vi "ChangePassword-Window.vi"(7 "PwdMgr":refnum<class "PwdMgr.lvclass">, 8 "error in (no error)":errorcluster, 11 "User Info":T1={"UserName"="", "Password"="", "Role"=enum."Admin"}) -> (0 "error out":errorcluster)   [LabVIEW 2020, in "Login-UI.lvlib"]
uses:
  Login-UI.lvlib
  _Typedef/User-Info.ctl
  _Typedef/User-Role.ctl
  PwdMgr/PwdMgr.lvclass
panel:
  in  "Exit":bool
  in  "Save":bool
  in  "密  码":string
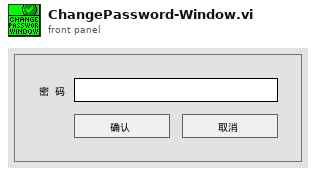
[diagram p1: front panel]
types:
  T1 = typedef "Login-UI.lvlib/User-Info.ctl" = cluster{"UserName":string, "Password":string, "Role":T2}
  T2 = typedef "Login-UI.lvlib/User-Role.ctl" = enum16{"INVALID", "Operator", "Engineer", "Admin", "Anonymous"}
  T3 = enum32{"Invalid", "Standard", "Closed", "Hidden", "Minimized", "Maximized"}
  T4 = enum32{"invalid app kind", "Development System", "Run Time System", "Student Edition", "Embedded LabVIEW", "Evaluation", "Custom"}
  T5 = cluster{"Core":cluster{"Current VI Reference":refnum<vi>, "Close Panel on Exit?":bool}, "Your Boolean data":bool, "Your string data":string, "User Info":T1}
  T6 = typedef "eventvkey.ctl" = enum16{"ASCII", "Enter", "Return", "Shift", "Ctrl", "Alt", "Cmd", "Opt", "Caps", "NumLock", "Clear", "Break", "Up", "Down", "Left", "Right", "Insert", "Delete", "Home", "End", "PageUp", "PageDown", "Escape", "Help", "Pause", "ScrollLock", "F1", "F2", "F3", "F4", "F5", "F6", "F7", "F8", "F9", "F10", "F11", "F12", "F13", "F14", "F15", "F16", "F17", "F18", "F19", "F20", "F21", "F22", "F23", "F24", "Play", "VolumeUp", "VolumeDown", "Mute", "Two Byte Char"}
  T7 = cluster{"Current VI Reference":refnum<vi>, "Close Panel on Exit?":bool}
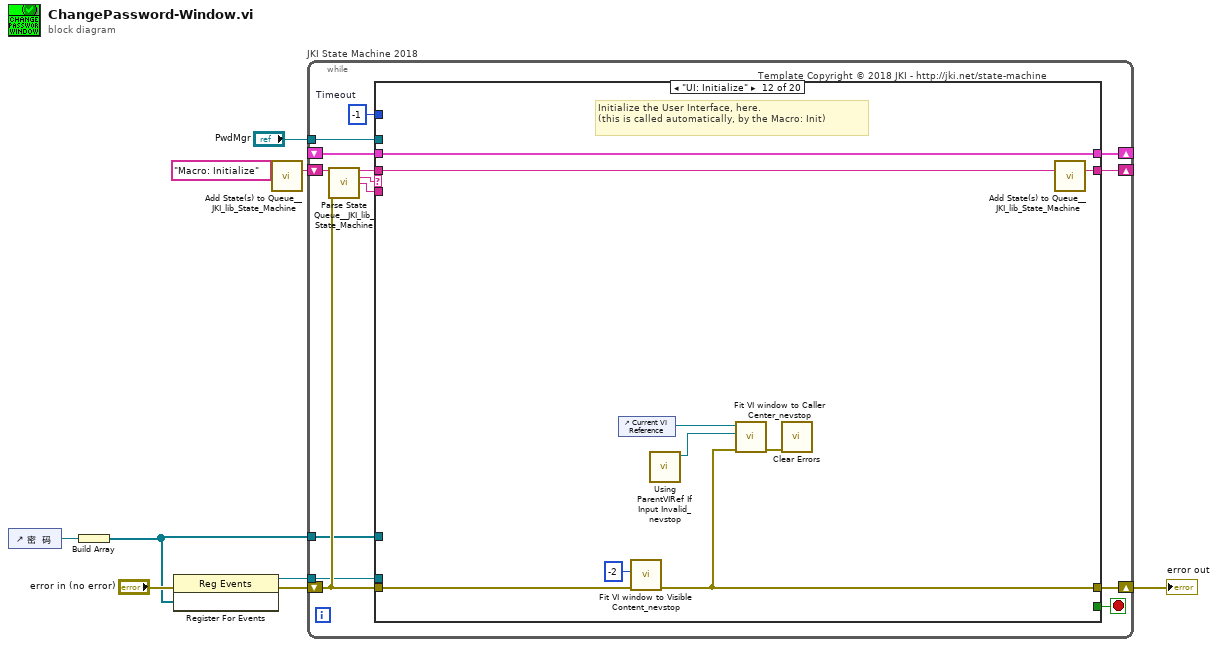
[diagram p0: block diagram]
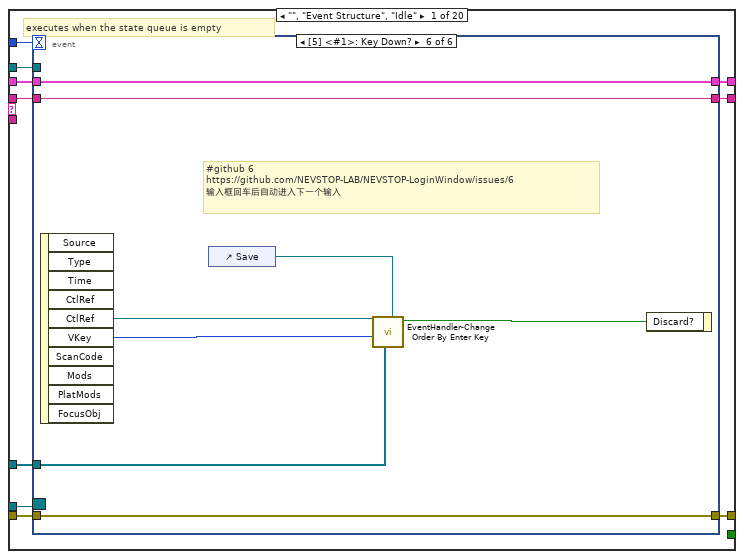
[diagram p2: hidden frame]
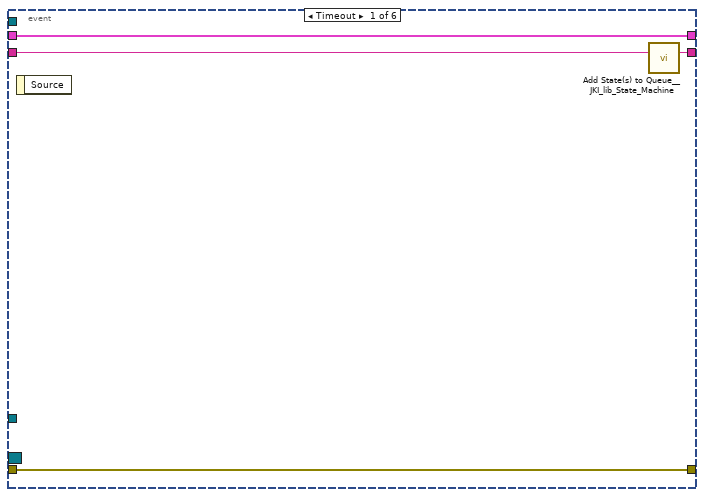
[diagram p3: hidden frame]
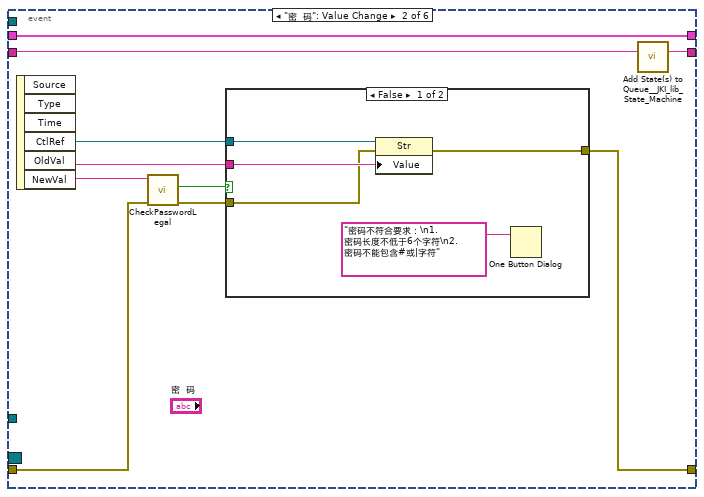
[diagram p4: hidden frame]
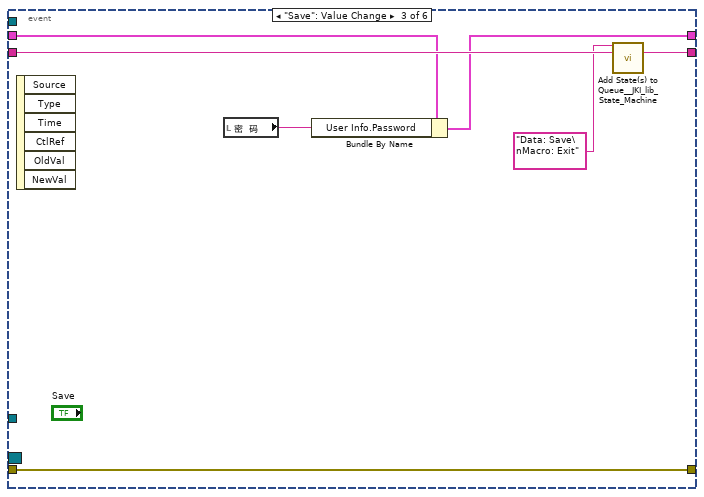
[diagram p6: hidden frame]
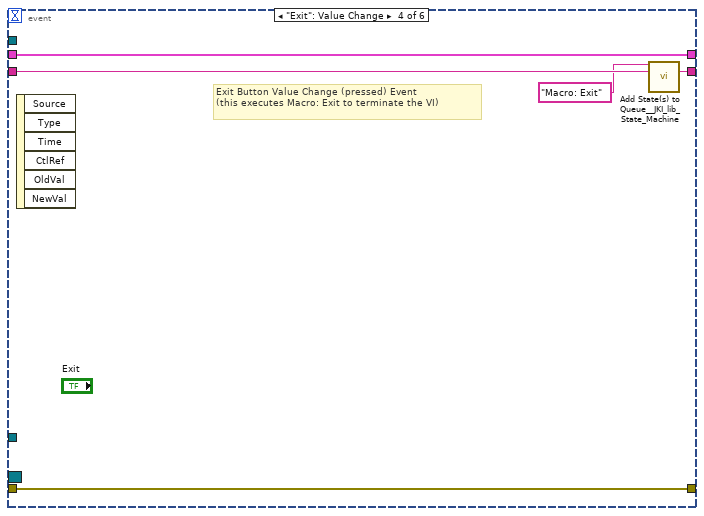
[diagram p7: hidden frame]
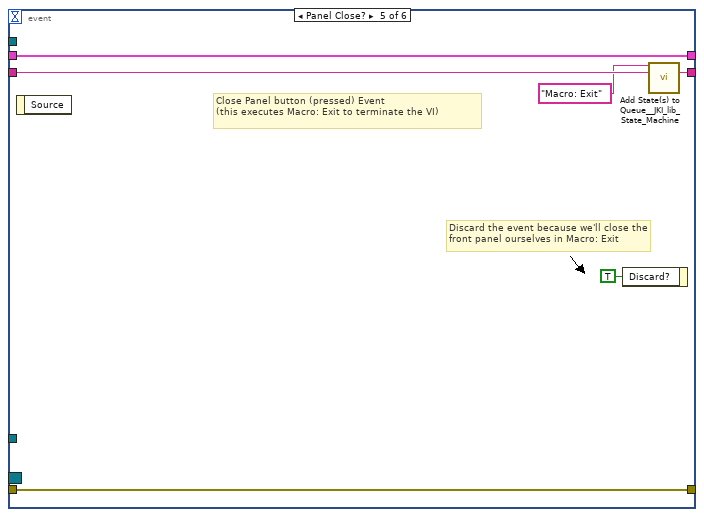
[diagram p8: hidden frame]
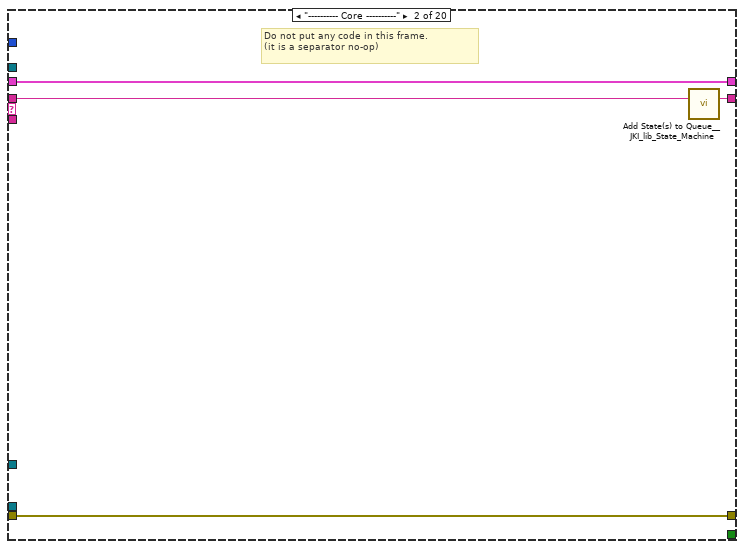
[diagram p9: hidden frame]
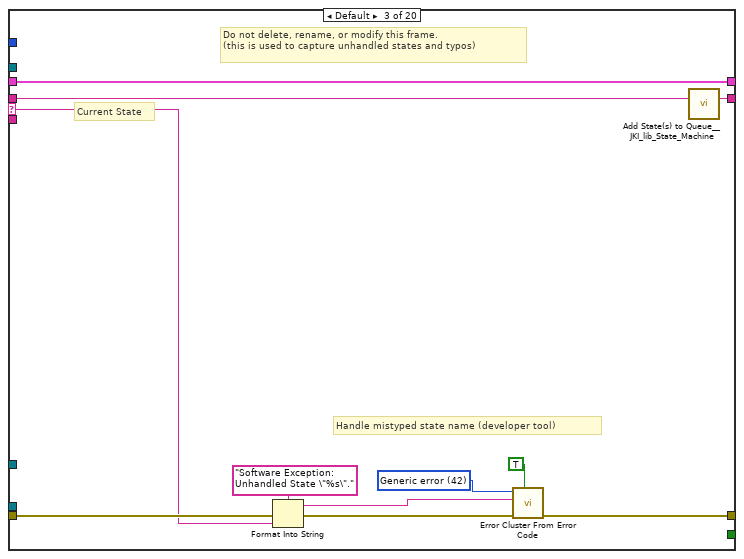
[diagram p10: hidden frame]
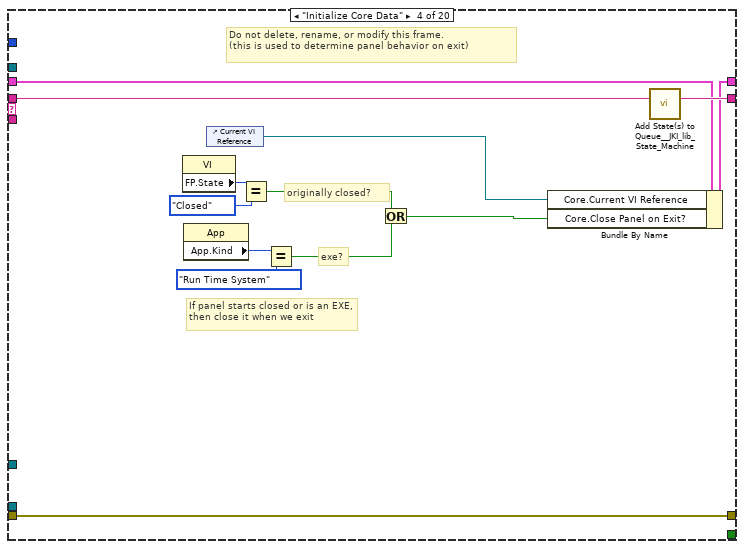
[diagram p11: hidden frame]
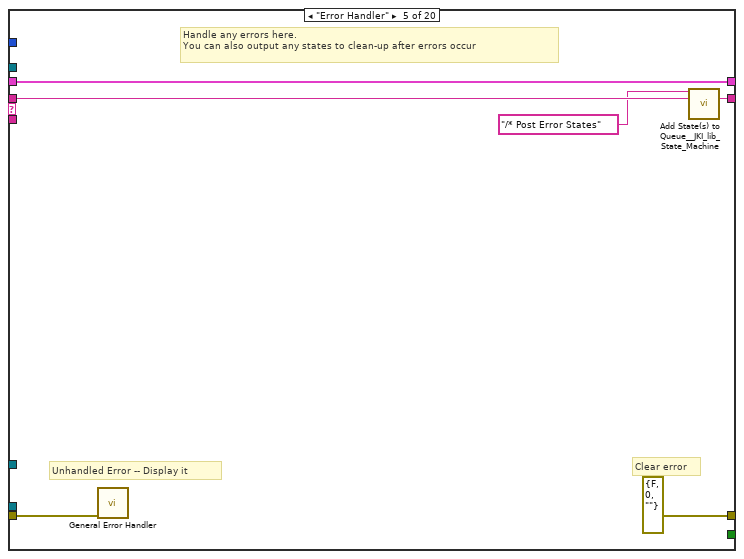
[diagram p12: hidden frame]
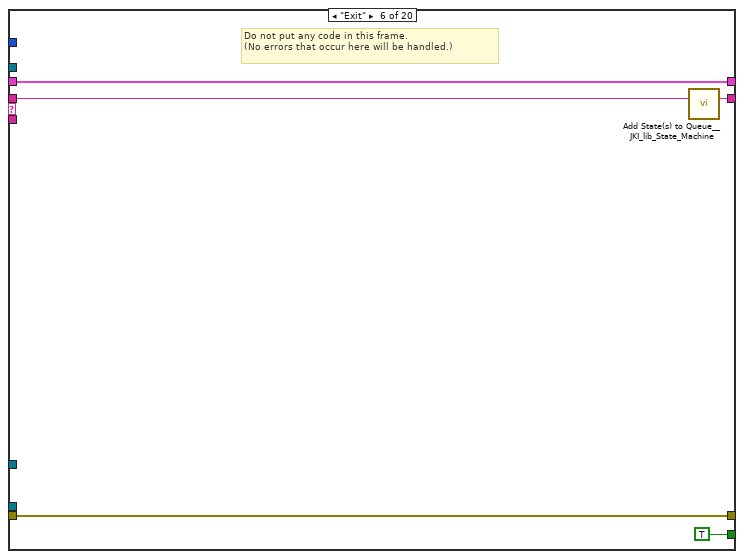
[diagram p13: hidden frame]
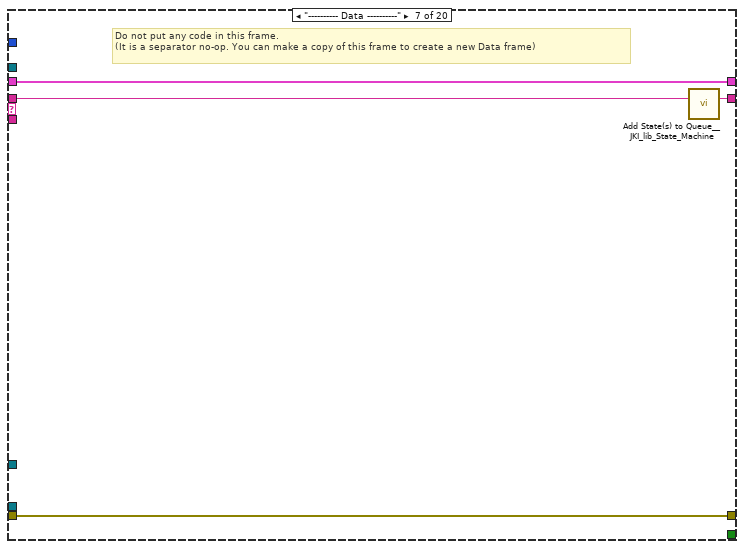
[diagram p14: hidden frame]
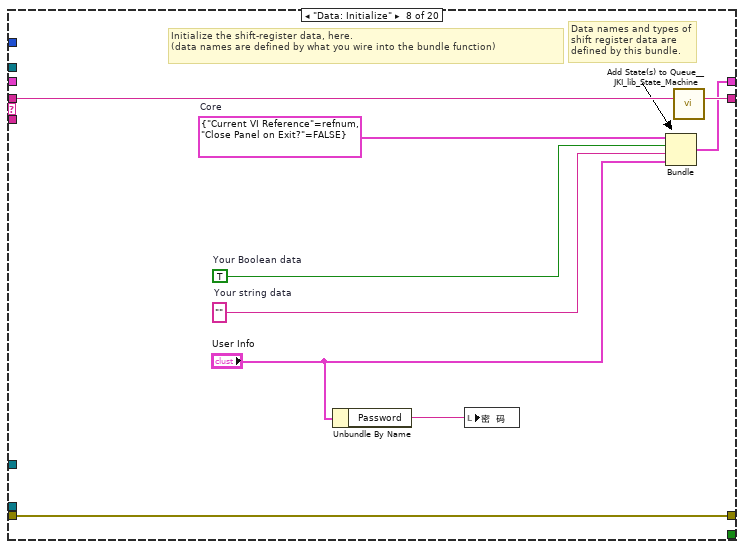
[diagram p15: hidden frame]
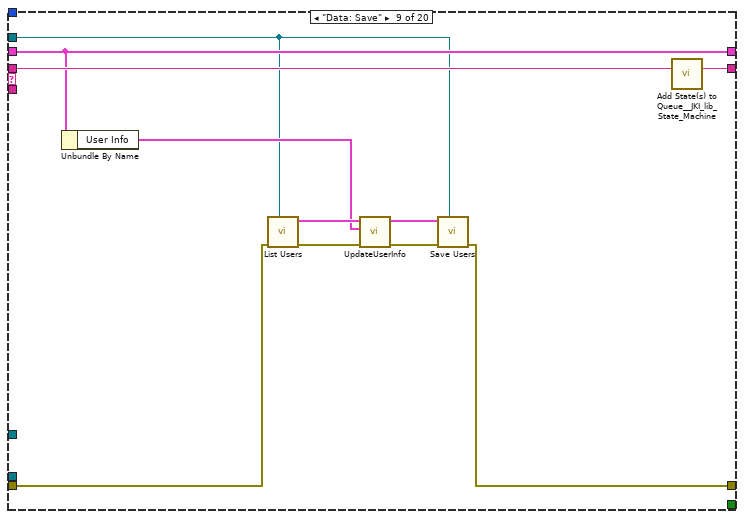
[diagram p16: hidden frame]
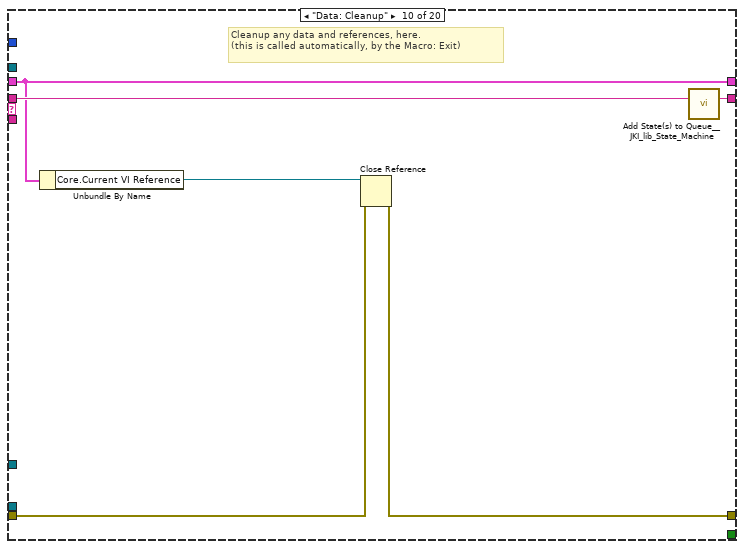
[diagram p17: hidden frame]
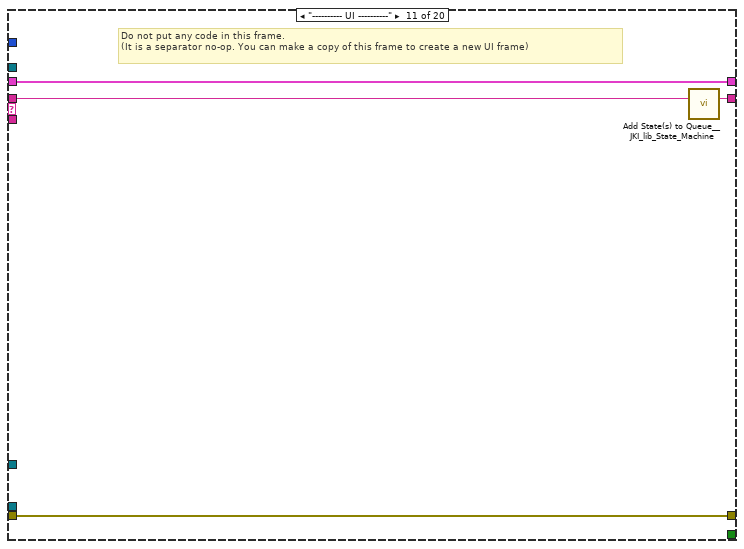
[diagram p18: hidden frame]
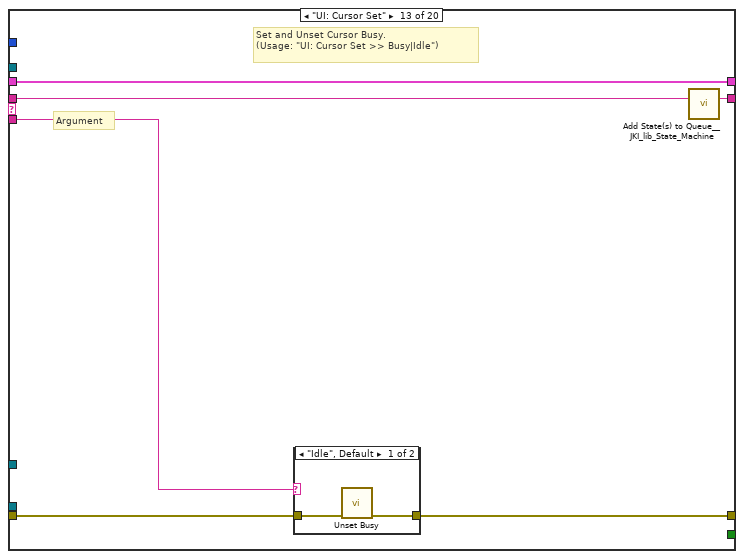
[diagram p19: hidden frame]
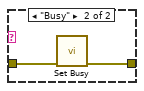
[diagram p20: hidden frame]
diagram:
  n1 = control-ref of="密  码"() -> (w3:refnum<vi>)
  n2 = Build Array(w3) -> (w2:refnum<vi>[])
  n3 = register-events(error in="error in (no error)", w2) -> (reference out=w4:refnum<event-registration>, error out=w5:errorcluster)  [unwired: 1 in]
  n4 = call <vilib>:"Add State(s) to Queue__JKI_lib_State_Machine.vi"("State(s) in (\"\")"="Macro: Initialize") -> ("States Out"=w9:string)  [unwired: 14 in]
  n5 = while "JKI State Machine 2018" {
    shift-right: [w16] -> _
    shift-left: _ -> [w15]
    shift-right: [w19] -> w6
    shift-left: w5 -> [w13]
    shift-right: [w18] -> _
    shift-left: w9 -> [w20]
    tunnel: w4 -> [w12]
    tunnel: w2 -> [w11]
    tunnel: "PwdMgr" -> [w10]
    stop <- w17 stop-if-true
    w14 = -1  # Timeout
    # "Template Copyright © 2018 JKI - http://jki.net/state-machine"
    n6 = call <vilib>:"Parse State Queue__JKI_lib_State_Machine.vi"("State Queue"=w20, "Error In (no error)"=w13) -> ("Remaining States"=w22:string, "Current State"=w23:string, "Arguments"=w21:string)  [unwired: 11 in]
    n7 = case shown="\"UI: Initialize\"" w23 {
      selector: w23 -> [_ _ w84 _ _ _ _ _ _ _ _ _ _ _ _ _ _ _ _ _]
      tunnel: w22 -> [w33 w83 w88 w107 w113 w118 w122 w131 w141 w148 w152 w161 w167 w178 w247 w252 w262 w266 w270 w274]
      tunnel: w21 -> [_ _ _ _ _ _ _ _ _ _ _ _ w162 w172 _ _ _ _ _ _]
      tunnel: w15 -> [w31 w80 w86 w100 w110 w116 w119 _ w133 w143 w149 w159 w165 w174 w244 w249 w259 w263 w267 w271]
      tunnel: [w30 w81 w90 w104 errorcluster {"status"=FALSE, "code"=0, "source"=""} ("error out") w115 w120 w128 w134 w144 w150 w153 w163 w175 w245 w250 w260 w264 w268 w272] -> w19
      tunnel: w13 -> [w29 w81 w89 w104 w109 w115 w120 w128 w135 w145 w150 w157 w164 w176 w245 w250 w260 w264 w268 w272]
      tunnel: [w32 w82 w87 w106 w112 w117 w121 w130 w142 w147 w151 w160 w166 w177 w246 w251 w261 w265 w269 w273] -> w18
      tunnel: [_ _ _ _ _ TRUE _ _ _ _ _ _ _ _ _ _ _ _ _ _] -> w17
      tunnel: [w28 w80 w86 w105 w110 w116 w119 w129 w133 w143 w149 w159 w165 w174 w244 w249 w259 w263 w267 w271] -> w16
      tunnel: w14 -> [w27 _ _ _ _ _ _ _ _ _ _ _ _ _ _ _ _ _ _ _]
      tunnel: w12 -> [w26 _ _ _ _ _ _ _ _ _ _ _ _ _ _ _ _ _ _ _]
      tunnel: w11 -> [w25 _ _ _ _ _ _ _ _ _ _ _ _ _ _ _ _ _ _ _]
      tunnel: w10 -> [w24 _ _ _ _ _ _ _ w132 _ _ _ _ _ _ _ _ _ _ _]
      frame "", "Event Structure", "Idle" {
        # "executes when the state queue is empty"
        n8 = event shown="[5] <#1>: Key Down?" {
          selector: w26 -> [_ _ _ _ _ _]
          dyn-events: _ -> [_ _ _ _ _ _]
          timeout: w27 -> [_ _ _ _ _ _]
          tunnel: w33 -> [w37 w41 w59 w65 w71 w73]
          tunnel: [w36 w42 w60 w64 w70 w73] -> w32
          tunnel: w31 -> [w34 w43 w57 w62 w68 w74]
          tunnel: [w35 w38 w55 w63 w69 w72] -> w30
          tunnel: w29 -> [w35 w40 w55 w63 w69 w72]
          tunnel: [w34 w43 w56 w62 w68 w74] -> w28
          tunnel: w25 -> [_ _ _ _ _ w76]
          tunnel: w24 -> [_ _ _ _ _ _]
          event Timeout {
            n9 = event-data() -> ()  [unwired: 1 in, 1 out]
            n10 = call <vilib>:"Add State(s) to Queue__JKI_lib_State_Machine.vi"("State(s) in (\"\")"=w37) -> ("States Out"=w36:string)  [unwired: 14 in]
          }
          event "密  码": Value Change {
            n11 = event-data() -> ("CtlRef"=w45:refnum<vi>, "OldVal"=w44:string, "NewVal"=w47:string)  [unwired: 1 in, 3 out]
            n12 = call "CheckPasswordLegal.vi"("error in (no error)"=w40, "Password"=w47) -> ("error out"=w39:errorcluster, "legal?"=w46:bool)  [unwired: 8 in]
            n13 = case shown="False" w46 {
              tunnel: w45 -> [w52 _]
              tunnel: w44 -> [w51 _]
              tunnel: w39 -> [w49 w53]
              tunnel: [w48 w53] -> w38
              frame False {
                n14 = property class="Str"(reference=w52, error in=w49, "Value"=w51) -> (error out=w48:errorcluster)  [unwired: 1 out]
                n15 = One Button Dialog(message="密码不符合要求：\n1.密码长度不低于6个字符\n2. 密码不能包含#或|字符") -> ()  [unwired: 1 in, 1 out]
              }
              frame True {
              }
            }
            n16 = call <vilib>:"Add State(s) to Queue__JKI_lib_State_Machine.vi"("State(s) in (\"\")"=w41) -> ("States Out"=w42:string)  [unwired: 14 in]
          }
          event "Save": Value Change {
            n17 = event-data() -> ()  [unwired: 1 in, 6 out]
            n18 = local read "密  码"() -> (w54:string)
            n19 = Bundle By Name(cluster=w57, "User Info.Password"=w54) -> (w56:T5)
            n20 = call <vilib>:"Add State(s) to Queue__JKI_lib_State_Machine.vi"("State(s) in Front (\"\")"="Data: Save\nMacro: Exit", "State(s) in (\"\")"=w59) -> ("States Out"=w60:string)  [unwired: 13 in]
          }
          event "Exit": Value Change {
            # "Exit Button Value Change (pressed) Event\n(this executes Macro: Exit to terminate the VI)"
            n21 = event-data() -> ()  [unwired: 1 in, 6 out]
            n22 = call <vilib>:"Add State(s) to Queue__JKI_lib_State_Machine.vi"("State(s) in Front (\"\")"="Macro: Exit", "State(s) in (\"\")"=w65) -> ("States Out"=w64:string)  [unwired: 13 in]
          }
          event Panel Close? {
            # "Discard the event because we'll close the front panel ourselves in Macro: Exit"
            # "Close Panel button (pressed) Event\n(this executes Macro: Exit to terminate the VI)"
            n23 = event-data() -> ()  [unwired: 1 in, 1 out]
            n24 = event-data("Discard?"=TRUE) -> ()  [unwired: 1 in, 1 out]
            n25 = call <vilib>:"Add State(s) to Queue__JKI_lib_State_Machine.vi"("State(s) in Front (\"\")"="Macro: Exit", "State(s) in (\"\")"=w71) -> ("States Out"=w70:string)  [unwired: 13 in]
          }
          event Key Down? {
            # "#github 6\nhttps://github.com/NEVSTOP-LAB/NEVSTOP-LoginWindow/issues/6\n输入框回车后自动进入下一个输入"
            n26 = event-data() -> ("CtlRef"=w79:refnum<vi>, "VKey"=w78:T6)  [unwired: 1 in, 8 out]
            n27 = control-ref of="Save"() -> (w77:refnum<vi>)
            n28 = call "EventHandler-Change Order By Enter Key.vi"("Next Ctrl"=w77, "Controls for changing order"=w76, "VKey"=w78, "Event Control"=w79) -> ("Discard?"=w75:bool)  [unwired: 7 in]
            n29 = event-data("Discard?"=w75) -> ()  [unwired: 1 in, 1 out]
          }
        }
      }
      frame "---------- Core ----------" {
        # "Do not put any code in this frame.\n(it is a separator no-op)"
        n30 = call <vilib>:"Add State(s) to Queue__JKI_lib_State_Machine.vi"("State(s) in (\"\")"=w83) -> ("States Out"=w82:string)  [unwired: 14 in]
      }
      frame Default {
        w93 = 42 items=["No error", "Argument error", "Memory is full", "Out of zone", "End of file", "File already open", "Generic file I/O error", "File not found", "File permission error", "Disk is full", "Duplicate path", "Too many files open", "System feature not enabled", "Resource file not found", "Cannot add resource", "Resource not found", "Image not found", "Image memory error", "Pen does not exist", "Config type invalid", "Config token not found", "Config parse error", "Config memory error", "Bad external code format", "Bad external code offset", "External code not present", "Null window", "Destroy window error", "Null menu", "Print aborted", "Bad print record", "Print driver error", "Windows error during printing", "Memory error during printing", "Print dialog error", "Generic print error", "Invalid device refnum", "Device not found", "Device parameter error", "Device unit error", "Cannot open device", "Device call aborted", "Generic error", "Cancelled by user", "Object ID too low", "Object ID too high", "Object not in heap", "Unknown heap", "Unknown object (invalid DefProc)", "Unknown object (DefProc not in table)", "Message out of range", "Invalid (null) method", "Unknown message", "Manager call not supported", "Bad address", "Network operation in progress", "Network operation timed out", "Connection is busy", "Network attribute not supported", "Network error", "Address in use", "System out of memory", "Connection aborted", "Connection refused", "Not connected", "Already connected", "Connection closed", "Initialization error (interapplication manager)", "Bad occurrence", "Wait on unbound occurrence handler", "Occurrence queue overflow", "Datalog type conflict", "Unused", "Unrecognized type (interapplication manager)", "Memory corrupt", "Failed to make temporary DLL", "Old CIN version", "Drag socket not found", "Failed to load drop-object", "Failed to register OLE object", "Failed to release OLE object", "Format specifier type mismatch", "Unknown format specifier", "Too few format specifiers", "Too many format specifiers", "Scan failed", "Newer CIN version", "Error converting to variant", "Runtime menu error", "Password tampered", "Variant attribute not found", "Incompatible variant data type", "Event data is not available", "Event Store is not present", "Occurrence is not found", "Event Queue is not created", "Event info is not available", "Refnum passed is NULL", "Error retrieving Class GUID", "Error retrieving CoClass GUID", "Error retrieving TypeLib GUID.", "Bad built application magic bytes.", "Specific driver is different from the specific driver associated with the Logical Name.", "There is no session opened to the class driver.", "Max Error", "MAX - Error with config objects", "MAX - Error loading configuration", "MAX - Group not supported"]
        # "Current State"
        # "Do not delete, rename, or modify this frame.\n(this is used to capture unhandled states and typos)"
        # "Handle mistyped state name (developer tool)"
        n31 = Format Into String(format string="Software Exception: Unhandled State \"%s\"." ("message"), error in=w89, w84) -> (resulting string=w92:string, error out=w91:errorcluster)  [unwired: 1 in]
        n32 = call <vilib>:"Error Cluster From Error Code.vi"("show call chain? (False)"=TRUE, "error in (no error)"=w91, "error message (\"\")"=w92, "error code (0)"=w93) -> ("error out"=w90:errorcluster)  [unwired: 5 in]
        n33 = call <vilib>:"Add State(s) to Queue__JKI_lib_State_Machine.vi"("State(s) in (\"\")"=w88) -> ("States Out"=w87:string)  [unwired: 14 in]
      }
      frame "Initialize Core Data" {
        # "Do not delete, rename, or modify this frame.\n(this is used to determine panel behavior on exit)"
        # "originally closed?"
        # "exe?"
        # "If panel starts closed or is an EXE, then close it when we exit"
        n34 = property class="VI"() -> ("FP.State"=w97:T3)  [unwired: 2 in, 2 out]
        n35 = property class="App"() -> ("App.Kind"=w103:T4)  [unwired: 2 in, 2 out]
        n36 = control-ref of="Current VI Reference"() -> (w98:refnum<vi>)
        n37 = Equal?(x=w97, y=T3."Closed" ("Front Panel Window:State")) -> (x = y?=w95:bool)
        n38 = Equal?(x=w103, y=T4."Run Time System" ("Application:Kind")) -> (x = y?=w101:bool)
        n39 = Or(x=w95, y=w101) -> (x .or. y?=w99:bool)
        n40 = Bundle By Name(cluster=w100, "Core.Current VI Reference"=w98, "Core.Close Panel on Exit?"=w99) -> (w105:T5)
        n41 = call <vilib>:"Add State(s) to Queue__JKI_lib_State_Machine.vi"("State(s) in (\"\")"=w107) -> ("States Out"=w106:string)  [unwired: 14 in]
      }
      frame "Error Handler" {
        # "Unhandled Error -- Display it"
        # "Handle any errors here.\nYou can also output any states to clean-up after errors occur"
        # "Clear error"
        n42 = call <vilib>:"General Error Handler.vi"("error in (no error)"=w109) -> ()  [unwired: 10 in, 5 out]
        n43 = call <vilib>:"Add State(s) to Queue__JKI_lib_State_Machine.vi"("State(s) in Front (\"\")"="/* Post Error States", "State(s) in (\"\")"=w113) -> ("States Out"=w112:string)  [unwired: 13 in]
      }
      frame "Exit" {
        # "Do not put any code in this frame.\n(No errors that occur here will be handled.)"
        n44 = call <vilib>:"Add State(s) to Queue__JKI_lib_State_Machine.vi"("State(s) in (\"\")"=w118) -> ("States Out"=w117:string)  [unwired: 14 in]
      }
      frame "---------- Data ----------" {
        # "Do not put any code in this frame.\n(It is a separator no-op. You can make a copy of this frame to create a new Data frame)"
        n45 = call <vilib>:"Add State(s) to Queue__JKI_lib_State_Machine.vi"("State(s) in (\"\")"=w122) -> ("States Out"=w121:string)  [unwired: 14 in]
      }
      frame "Data: Initialize" {
        w125 = T7 {"Current VI Reference"=refnum, "Close Panel on Exit?"=FALSE}  # Core
        w127 = TRUE  # Your Boolean data
        w126 = ""  # Your string data
        # "Data names and types of shift register data are defined by this bundle."
        # "Initialize the shift-register data, here.\n(data names are defined by what you wire into the bundle function)"
        n46 = Unbundle By Name("User Info") -> ("Password"=w123:string)
        n47 = local write "密  码"(w123) -> ()
        n48 = Bundle("Core"=w125, "Your Boolean data"=w127, "Your string data"=w126, "User Info"="User Info") -> (w129:T5)  [unwired: 1 in]
        n49 = call <vilib>:"Add State(s) to Queue__JKI_lib_State_Machine.vi"("State(s) in (\"\")"=w131) -> ("States Out"=w130:string)  [unwired: 14 in]
      }
      frame "Data: Save" {
        n50 = Unbundle By Name(w133) -> ("User Info"=w139:T1)
        n51 = call-dynamic "List Users.vi"("PwdMgr in"=w132, "error in (no error)"=w135) -> ("error out"=w138:errorcluster, "Array"=w140:T1[])  [unwired: 8 in]
        n52 = call "UpdateUserInfo.vi"("error in"=w138, "User"=w139, "User List"=w140) -> ("error out"=w136:errorcluster, "User List"=w137:T1[])  [unwired: 7 in]
        n53 = call-dynamic "Save Users.vi"("PwdMgr in"=w132, "error in (no error)"=w136, "Array"=w137) -> ("error out"=w134:errorcluster)  [unwired: 8 in]
        n54 = call <vilib>:"Add State(s) to Queue__JKI_lib_State_Machine.vi"("State(s) in (\"\")"=w141) -> ("States Out"=w142:string)  [unwired: 14 in]
      }
      frame "Data: Cleanup" {
        # "Cleanup any data and references, here.\n(this is called automatically, by the Macro: Exit)"
        n55 = Unbundle By Name(w143) -> ("Core.Current VI Reference"=w146:refnum<vi>)
        n56 = Close Reference(reference=w146, error in (no error)=w145) -> (error out=w144:errorcluster)
        n57 = call <vilib>:"Add State(s) to Queue__JKI_lib_State_Machine.vi"("State(s) in (\"\")"=w148) -> ("States Out"=w147:string)  [unwired: 14 in]
      }
      frame "---------- UI ----------" {
        # "Do not put any code in this frame.\n(It is a separator no-op. You can make a copy of this frame to create a new UI frame)"
        n58 = call <vilib>:"Add State(s) to Queue__JKI_lib_State_Machine.vi"("State(s) in (\"\")"=w152) -> ("States Out"=w151:string)  [unwired: 14 in]
      }
      frame "UI: Initialize" {
        # "Initialize the User Interface, here.\n(this is called automatically, by the Macro: Init)"
        n59 = control-ref of="Current VI Reference"() -> (w155:refnum<vi>)
        n60 = call <userlib>:"Fit VI window to Visible Content_nevstop.vi"("error in (no error)"=w157, "border spacing (2 px)"=-2) -> ("error out"=w153:errorcluster)  [unwired: 4 in, 1 out]
        n61 = call <userlib>:"Using ParentVIRef If Input Invalid_nevstop.vi"() -> ("VI Ref"=w154:refnum<vi>)  [unwired: 6 in, 1 out]
        n62 = call <userlib>:"Fit VI window to Caller Center_nevstop.vi"("Error In"=w153, "Background VI Ref (Callee's Caller)"=w154, "VI Ref (calling VI)"=w155) -> ("Error Out"=w156:errorcluster)  [unwired: 3 in, 1 out]
        n63 = call <vilib>:"Clear Errors.vi"("error in (no error)"=w156) -> ()  [unwired: 5 in, 2 out]
        n64 = call <vilib>:"Add State(s) to Queue__JKI_lib_State_Machine.vi"("State(s) in (\"\")"=w161) -> ("States Out"=w160:string)  [unwired: 14 in]
      }
      frame "UI: Cursor Set" {
        # "Argument"
        # "Set and Unset Cursor Busy.\n(Usage: \"UI: Cursor Set >> Busy|Idle\")"
        n65 = case shown="\"Idle\", Default" w162 {
          tunnel: w164 -> [w169 w171]
          tunnel: [w168 w170] -> w163
          frame "Idle", Default {
            n66 = call <vilib>:"Unset Busy.vi"("error in (no error)"=w169) -> ("error out"=w168:errorcluster)  [unwired: 10 in]
          }
          frame "Busy" {
            n67 = call <vilib>:"Set Busy.vi"("error in (no error)"=w171) -> ("error out"=w170:errorcluster)  [unwired: 9 in, 1 out]
          }
        }
        n68 = call <vilib>:"Add State(s) to Queue__JKI_lib_State_Machine.vi"("State(s) in (\"\")"=w167) -> ("States Out"=w166:string)  [unwired: 14 in]
      }
      frame "UI: Front Panel State" {
        # "Argument"
        # "Set Front Panel Open or Closed\n(Usage: \"UI: Front Panel State >> Open|Close\")"
        n69 = Unbundle By Name(w174) -> ("Core.Current VI Reference"=w173:refnum<vi>)
        n70 = case shown="\"Minimize\", \"Minimized\"" w172 {
          tunnel: w176 -> [w184 w199 w210 w223 w236]
          tunnel: [w186 w200 w212 w225 w238] -> w175
          tunnel: w173 -> [w185 w197 w211 w224 w237]
          frame "Open", "Standard", Default {
            w179 = T3."Standard" ("State")
            n71 = property class="VI"(reference=w185, error in=w184) -> (reference out=w182:refnum<vi>, error out=w183:errorcluster, "FP.State"=w181:T3)
            n72 = Not Equal?(x=w181, y=w179) -> (x != y?=w180:bool)
            n73 = case shown="True" w180 {
              tunnel: [w190 w192] -> w186
              tunnel: w183 -> [w189 w192]
              tunnel: w182 -> [w188 _]
              tunnel: w179 -> [w187 _]
              frame True {
                n74 = invoke class="VI" method="FP.Open"(reference=w188, error in=w189, "Activate"=TRUE, "State"=w187) -> (error out=w190:errorcluster)  [unwired: 1 in, 4 out]
              }
              frame False {
              }
            }
          }
          frame "Close", "Closed" {
            n75 = property class="VI"(reference=w197, error in=w199) -> (reference out=w196:refnum<vi>, error out=w198:errorcluster, "FP.State"=w194:T3)
            n76 = Not Equal?(x=w194, y=T3."Closed" ("Front Panel Window:State")) -> (x != y?=w193:bool)
            n77 = case shown="True" w193 {
              tunnel: [w201 w204] -> w200
              tunnel: w198 -> [w201 w203]
              tunnel: w196 -> [_ w202]
              frame False {
              }
              frame True {
                n78 = invoke class="VI" method="FP.Close"(reference=w202, error in=w203) -> (error out=w204:errorcluster)  [unwired: 1 in, 2 out]
              }
            }
          }
          frame "Hidden", "Hide" {
            w205 = T3."Hidden" ("State")
            n79 = property class="VI"(reference=w211, error in=w210) -> (reference out=w208:refnum<vi>, error out=w209:errorcluster, "FP.State"=w207:T3)
            n80 = Not Equal?(x=w207, y=w205) -> (x != y?=w206:bool)
            n81 = case shown="True" w206 {
              tunnel: [w216 w217] -> w212
              tunnel: w209 -> [w215 w217]
              tunnel: w208 -> [w214 _]
              tunnel: w205 -> [w213 _]
              frame True {
                n82 = invoke class="VI" method="FP.Open"(reference=w214, error in=w215, "State"=w213) -> (error out=w216:errorcluster)  [unwired: 2 in, 4 out]
              }
              frame False {
              }
            }
          }
          frame "Minimize", "Minimized" {
            w218 = T3."Minimized" ("State")
            n83 = property class="VI"(reference=w224, error in=w223) -> (reference out=w221:refnum<vi>, error out=w222:errorcluster, "FP.State"=w220:T3)
            n84 = Not Equal?(x=w220, y=w218) -> (x != y?=w219:bool)
            n85 = case shown="True" w219 {
              tunnel: [w229 w230] -> w225
              tunnel: w222 -> [w228 w230]
              tunnel: w221 -> [w227 _]
              tunnel: w218 -> [w226 _]
              frame True {
                n86 = invoke class="VI" method="FP.Open"(reference=w227, error in=w228, "State"=w226) -> (error out=w229:errorcluster)  [unwired: 2 in, 4 out]
              }
              frame False {
              }
            }
          }
          frame "Maximize", "Maximized" {
            w231 = T3."Maximized" ("State")
            n87 = property class="VI"(reference=w237, error in=w236) -> (reference out=w234:refnum<vi>, error out=w235:errorcluster, "FP.State"=w233:T3)
            n88 = Not Equal?(x=w233, y=w231) -> (x != y?=w232:bool)
            n89 = case shown="True" w232 {
              tunnel: [w242 w243] -> w238
              tunnel: w235 -> [w241 w243]
              tunnel: w234 -> [w240 _]
              tunnel: w231 -> [w239 _]
              frame True {
                n90 = invoke class="VI" method="FP.Open"(reference=w240, error in=w241, "State"=w239) -> (error out=w242:errorcluster)  [unwired: 2 in, 4 out]
              }
              frame False {
              }
            }
          }
        }
        n91 = call <vilib>:"Add State(s) to Queue__JKI_lib_State_Machine.vi"("State(s) in (\"\")"=w178) -> ("States Out"=w177:string)  [unwired: 14 in]
      }
      frame "---------- Macro ----------" {
        # "Do not put any code in this frame.\n(It is a separator no-op. You can make a copy of this frame to create a new Macro frame)"
        n92 = call <vilib>:"Add State(s) to Queue__JKI_lib_State_Machine.vi"("State(s) in (\"\")"=w247) -> ("States Out"=w246:string)  [unwired: 14 in]
      }
      frame "Macro: Initialize" {
        w248 = "Data: Initialize\nInitialize Core Data\nUI: Initialize\nUI: Front Panel State >> Open"  # Data: Initialize Initialize Core Data UI: Initialize UI: Front Panel State >> Open
        # "Initialization Macro\n(This is called once, when the VI starts)"
        n93 = call <vilib>:"Add State(s) to Queue__JKI_lib_State_Machine.vi"("State(s) in Front (\"\")"=w248, "State(s) in (\"\")"=w252) -> ("States Out"=w251:string)  [unwired: 13 in]
      }
      frame "Macro: Exit" {
        # "Exit Macro\n(This is called once, when the VI exits)"
        n94 = Unbundle By Name(w259) -> ("Core.Close Panel on Exit?"=w258:bool)
        n95 = Select(t="UI: Front Panel State >> Close", s=w258, f="") -> (s? t:f=w255:string)
        n96 = call <vilib>:"Add State(s) to Queue__JKI_lib_State_Machine.vi"("State(s) in (\"\")"=w255, "State(s) at Back (\"\")"="Data: Cleanup\nExit") -> ("States Out"=w253:string)  [unwired: 13 in]
        n97 = call <vilib>:"Add State(s) to Queue__JKI_lib_State_Machine.vi"("State(s) in Front (\"\")"=w253, "State(s) in (\"\")"=w262) -> ("States Out"=w261:string)  [unwired: 13 in]
      }
      frame "---------- New Category ----------" {
        # "Template Separator\n(You can make a copy of, or modify, this frame)"
        n98 = call <vilib>:"Add State(s) to Queue__JKI_lib_State_Machine.vi"("State(s) in (\"\")"=w266) -> ("States Out"=w265:string)  [unwired: 14 in]
      }
      frame "New Category: 1" {
        # "Your code here.\n(You can make a copy of, or modify, this frame)"
        n99 = call <vilib>:"Add State(s) to Queue__JKI_lib_State_Machine.vi"("State(s) in (\"\")"=w270) -> ("States Out"=w269:string)  [unwired: 14 in]
      }
      frame "New Category: 2" {
        # "Your code here.\n(You can make a copy of, or modify, this frame)"
        n100 = call <vilib>:"Add State(s) to Queue__JKI_lib_State_Machine.vi"("State(s) in (\"\")"=w274) -> ("States Out"=w273:string)  [unwired: 14 in]
      }
    }
  }
  "error out" <- w6
